vi "QMH Main.vi"() -> ()   [LabVIEW 2021]
doc: "Demonstrates the fundamentals of the Queued Message Handler design pattern in LabVIEW. A queued message handler, in its simplest form, is composed of two loops. The Event Handling Loop responds to user interface events by enqueuing \"messages\" on a message queue. These messages are dequeued in the Message Handling Loop. Note that the Message Handling Loop is also capable of sending messages to itself."
uses:
  <vilib>/MakerHub/PS4-Controller/Private/Type Defs/Indicators/Controller.ctl
  <vilib>/MakerHub/PS4-Controller/Private/Type Defs/Indicators/Square.ctl
  <vilib>/MakerHub/PS4-Controller/Private/Type Defs/Indicators/X.ctl
  <vilib>/MakerHub/PS4-Controller/Private/Type Defs/Indicators/Circle.ctl
  <vilib>/MakerHub/PS4-Controller/Private/Type Defs/Indicators/Triangle.ctl
  <vilib>/MakerHub/PS4-Controller/Private/Type Defs/Indicators/L1.ctl
  <vilib>/MakerHub/PS4-Controller/Private/Type Defs/Indicators/R1.ctl
  <vilib>/MakerHub/PS4-Controller/Private/Type Defs/Indicators/Share.ctl
  <vilib>/MakerHub/PS4-Controller/Private/Type Defs/Indicators/Options.ctl
  <vilib>/MakerHub/PS4-Controller/Private/Type Defs/Indicators/PS.ctl
  <vilib>/MakerHub/PS4-Controller/Private/Type Defs/Indicators/Pad_Button.ctl
  <vilib>/MakerHub/PS4-Controller/Private/Type Defs/Indicators/Dpad.ctl
  <vilib>/MakerHub/PS4-Controller/Private/Type Defs/Indicators/Slider.ctl
  C:/Program Files (x86)/National Instruments/LabVIEW 2021/examples/Design Patterns/Queued Message Handler/support/QMH Fundamentals - Message Cluster.ctl
  Classes/Actuation/Spring Motor/Spring Motor.lvclass
  Classes/Actuation/Motor/DC Motor.lvclass
  Classes/Sensing/IMU/IMU.lvclass
  Classes/Sensing/Ultrasonic Sensor/Ultrasonic Sensor.lvclass
  <vilib>/Utility/error.llb/Error Cluster From Error Code.vi
  <vilib>/MakerHub/PS4-Controller/Public/Open First Controller.vi
  <vilib>/ErrorRing/Error Ring.xnode
  Classes/Communication/Comm/Comm.lvclass
  <vilib>/MakerHub/PS4-Controller/LMH-PS4.lvlib
panel:
  out "PS4 Controller":T1={"Square Button"=FALSE, "X Button"=FALSE, "Circle Button"=FALSE, "Triangle Button"=FALSE, "L1"=FALSE, "R1"=FALSE, "Share Button"=FALSE, "Options Button"=FALSE, "PS Button"=FALSE, "Pad Button"=FALSE, "D-Pad"=5, "L2"=0, "R2"=0, "Thumbstick_Left"={[], []}, "Thumbstick_Right"={[], []}} {"R2" scale=-32768.0..32767.0; "L2" scale=-32768.0..32767.0}
  out "Checkbox":bool
  out "error out":errorcluster
  in  "Motor B Enable":bool
  in  "Motor B PWM":i16(slide) scale=0.0..255.0
  in  "Motor A Enable":bool
  in  "Motor A PWM":i16(slide) scale=0.0..255.0
  in  "Spring Motor Enable":bool
  in  "Spring Motor PWM":i16(slide) scale=0.0..180.0
  out "Display Message":string
  in  "Stop":bool
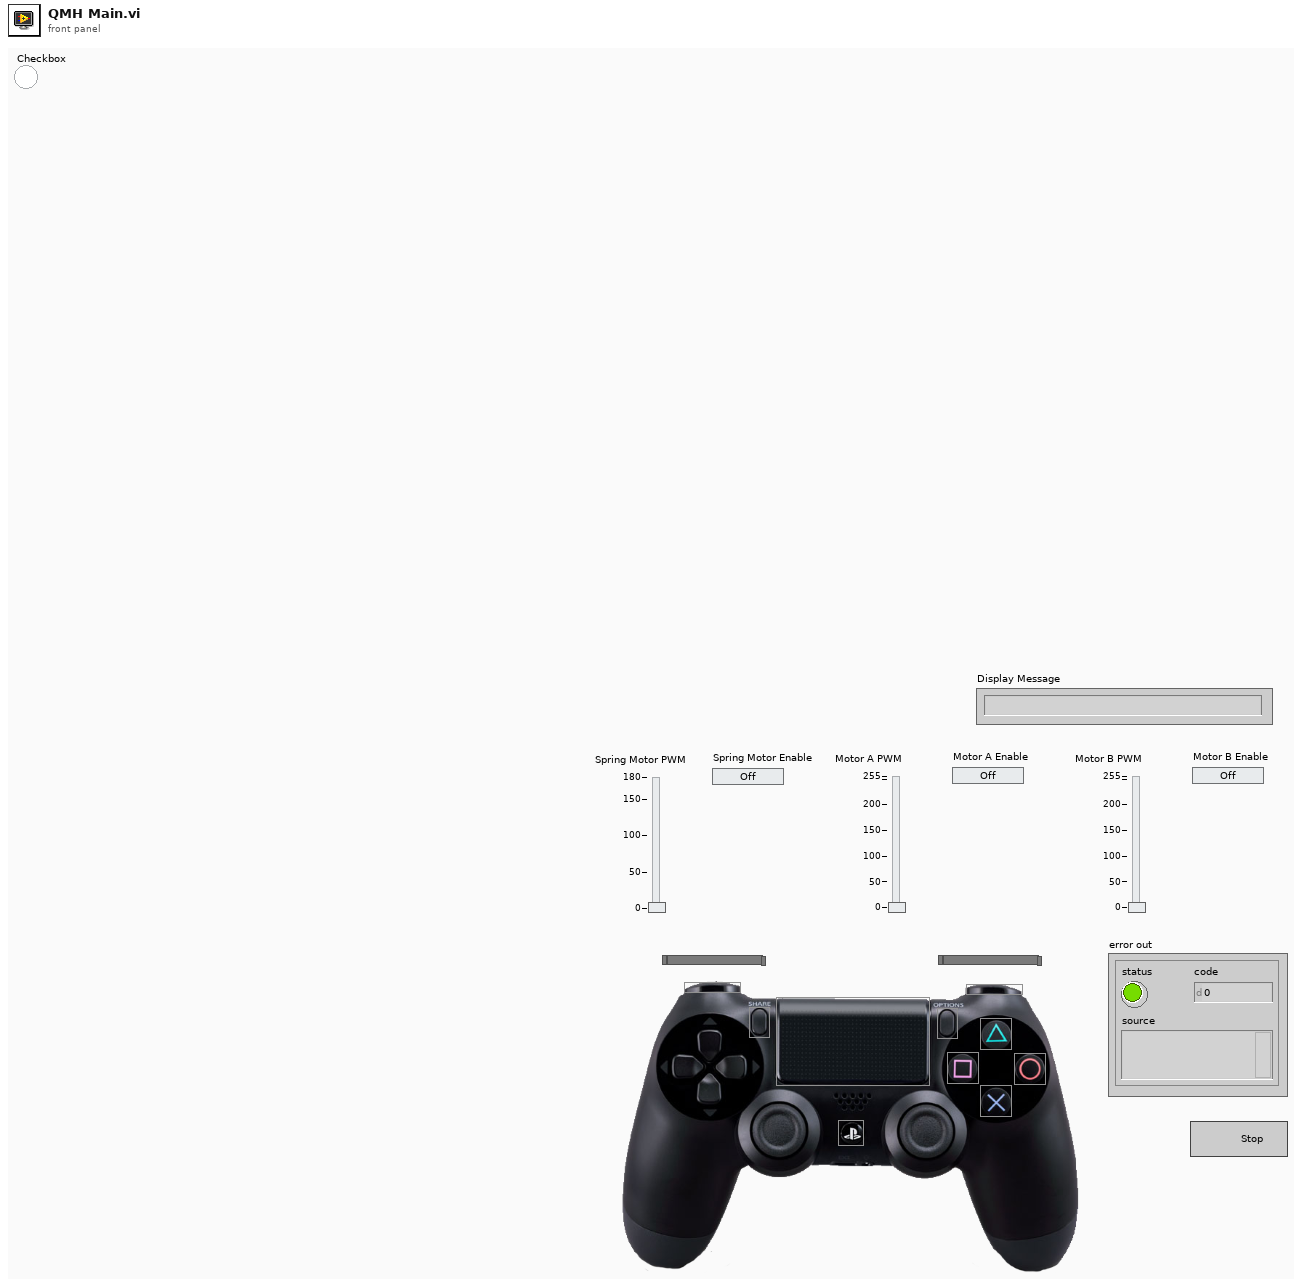
[diagram p1: front panel]
types:
  T1 = typedef "LMH-PS4.lvlib/Controller.ctl" = cluster{"Square Button":T2, "X Button":T3, "Circle Button":T4, "Triangle Button":T5, "L1":T6, "R1":T7, "Share Button":T8, "Options Button":T9, "PS Button":T10, "Pad Button":T11, "D-Pad":T12, "L2":T13, "R2":T13, "Thumbstick_Left":cluster{i32[], i32[]}, "Thumbstick_Right":cluster{i32[], i32[]}}
  T2 = typedef "LMH-PS4.lvlib/Square.ctl" = bool
  T3 = typedef "LMH-PS4.lvlib/X.ctl" = bool
  T4 = typedef "LMH-PS4.lvlib/Circle.ctl" = bool
  T5 = typedef "LMH-PS4.lvlib/Triangle.ctl" = bool
  T6 = typedef "LMH-PS4.lvlib/L1.ctl" = bool
  T7 = typedef "LMH-PS4.lvlib/R1.ctl" = bool
  T8 = typedef "LMH-PS4.lvlib/Share.ctl" = bool
  T9 = typedef "LMH-PS4.lvlib/Options.ctl" = bool
  T10 = typedef "LMH-PS4.lvlib/PS.ctl" = bool
  T11 = typedef "LMH-PS4.lvlib/Pad_Button.ctl" = bool
  T12 = typedef "LMH-PS4.lvlib/Dpad.ctl" = u16
  T13 = typedef "LMH-PS4.lvlib/Slider.ctl" = i32
  T14 = typedef "QMH Fundamentals - Message Cluster.ctl" = cluster{"Message":string, "Message Data":variant}
  T15 = typedef "LMH-PS4.lvlib/PS4 Controller Ref.ctl" = cluster{"Controller Ref":refnum<k1>, "Worker Ref":refnum<vi>, "PS4 Events Ref":refnum<event-registration>}
  T16 = typedef "LMH-PS4.lvlib/Axis.ctl" = cluster{"Left Thumbstick":cluster{"X Axis":i32, "Y Axis":i32}, "Right Thumbstick":cluster{"X Axis":i32, "Y Axis":i32}, "L2":i32, "R2":i32, "D-Pad":T17}
  T17 = typedef "LMH-PS4.lvlib/DPad Enum.ctl" = enum16{"Idle", "Up", "Up / Right", "Right", "Down / Right", "Down", "Down / Left", "Left", "Up / Left"}
  T18 = typedef "LMH-PS4.lvlib/Buttons.ctl" = cluster{"Square":bool, "X":bool, "Circle":bool, "Triangle":bool, "L1":bool, "R1":bool, "L2":bool, "R2":bool, "Share":bool, "Options":bool, "Left Thumbstick":bool, "Right Thumbstick":bool, "Playstation Button":bool, "Pad":bool}
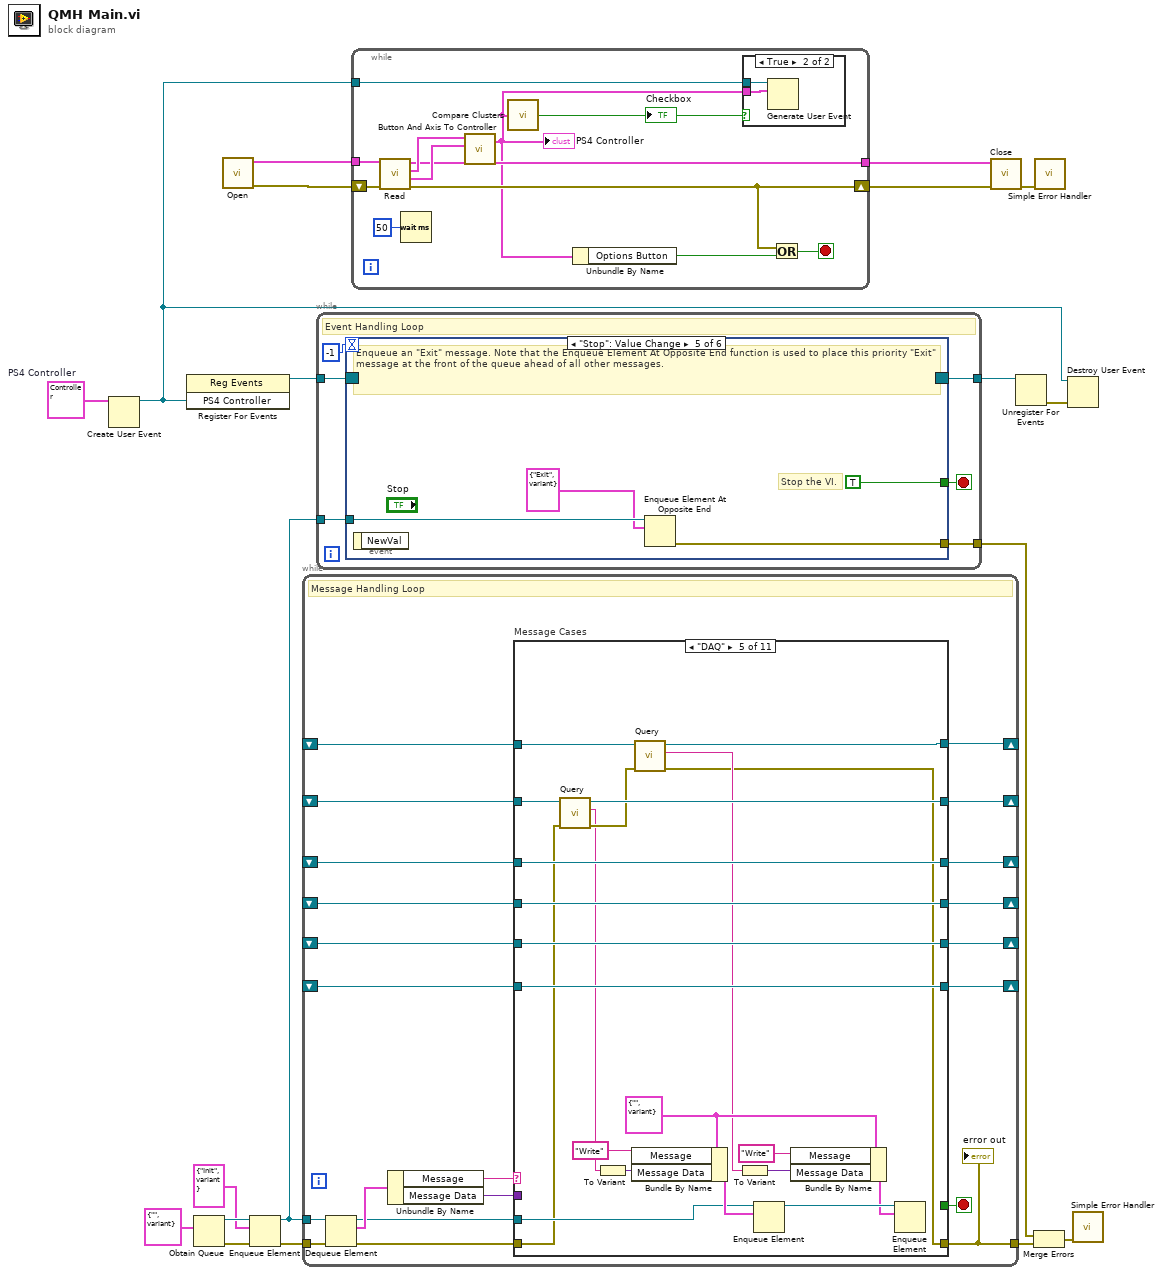
[diagram p0: block diagram]
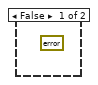
[diagram p2: hidden frame]
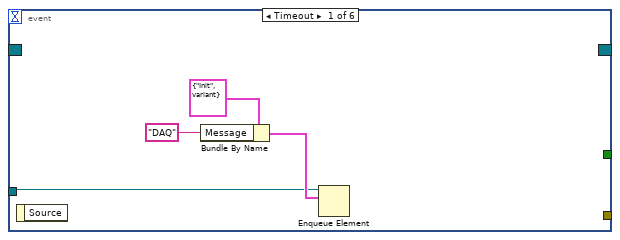
[diagram p3: hidden frame]
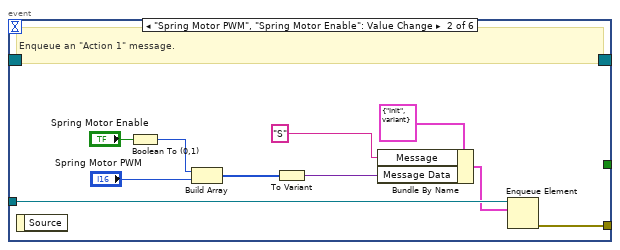
[diagram p4: hidden frame]
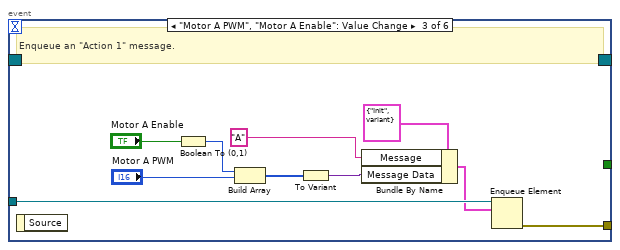
[diagram p5: hidden frame]
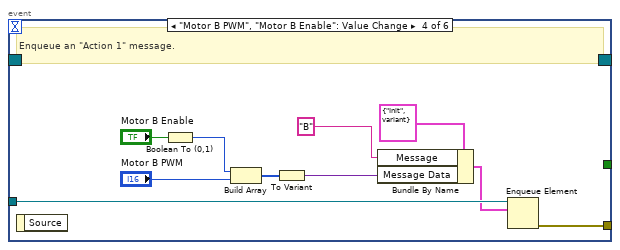
[diagram p6: hidden frame]
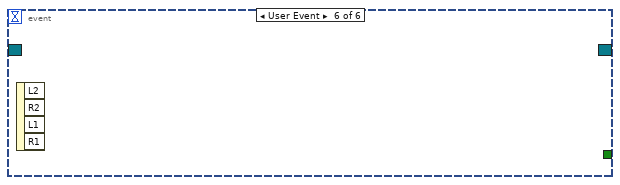
[diagram p7: hidden frame]
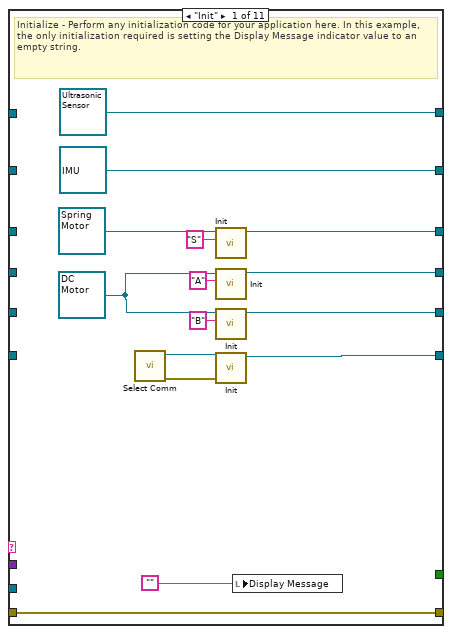
[diagram p8: hidden frame]
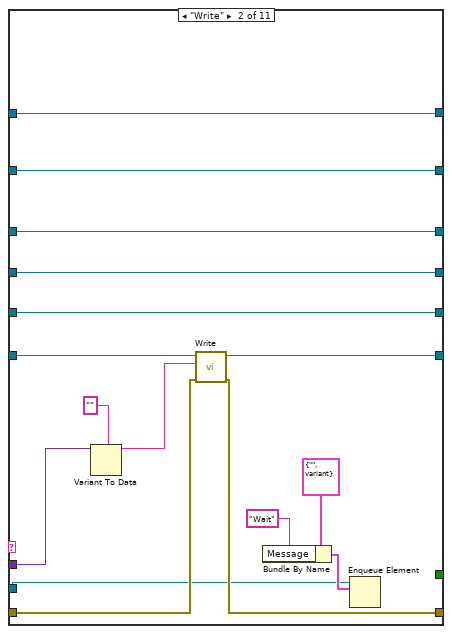
[diagram p9: hidden frame]
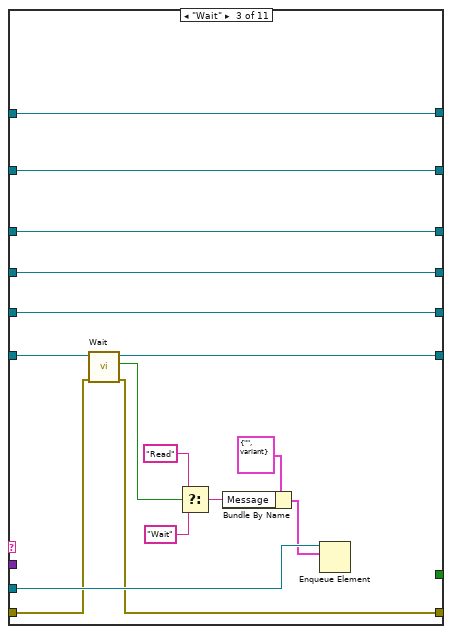
[diagram p10: hidden frame]
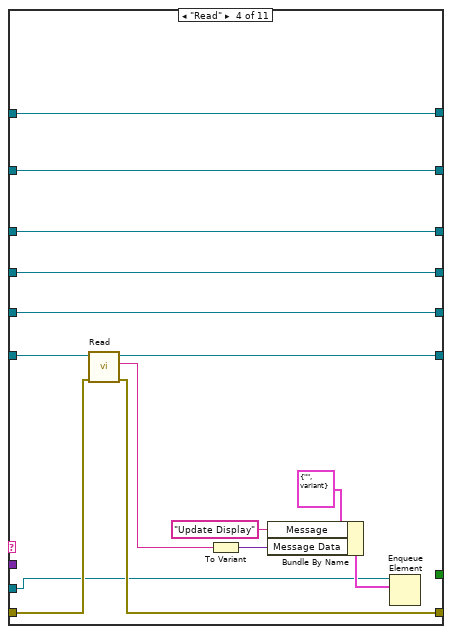
[diagram p11: hidden frame]
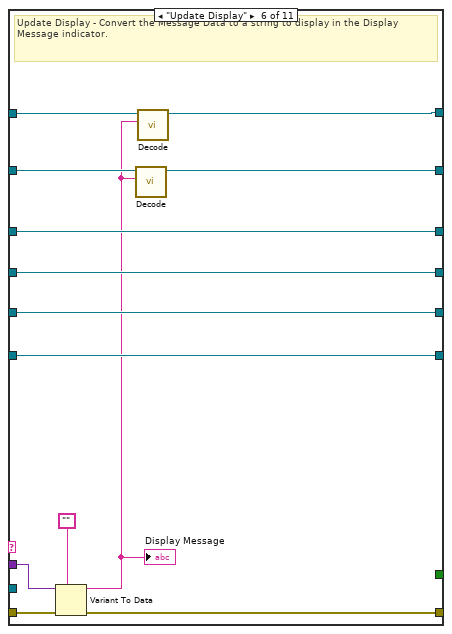
[diagram p12: hidden frame]
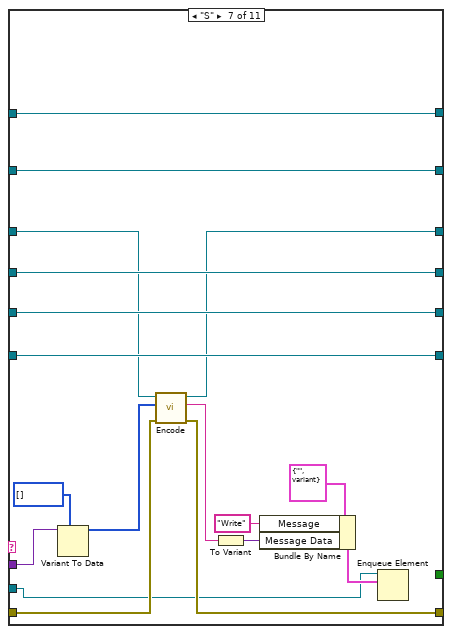
[diagram p13: hidden frame]
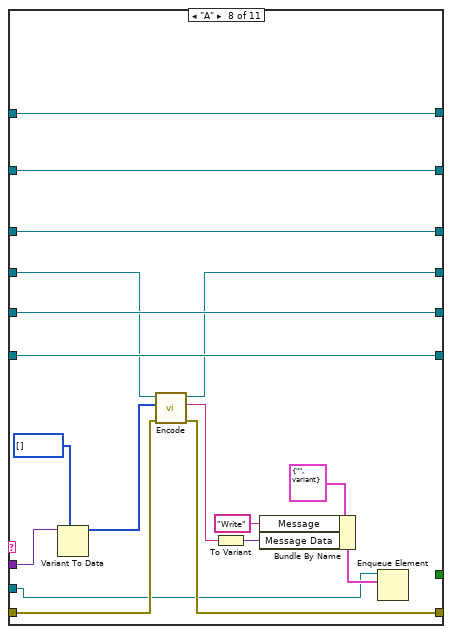
[diagram p14: hidden frame]
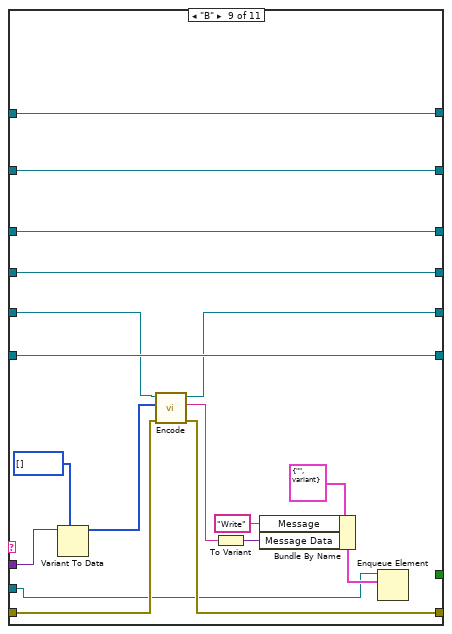
[diagram p15: hidden frame]
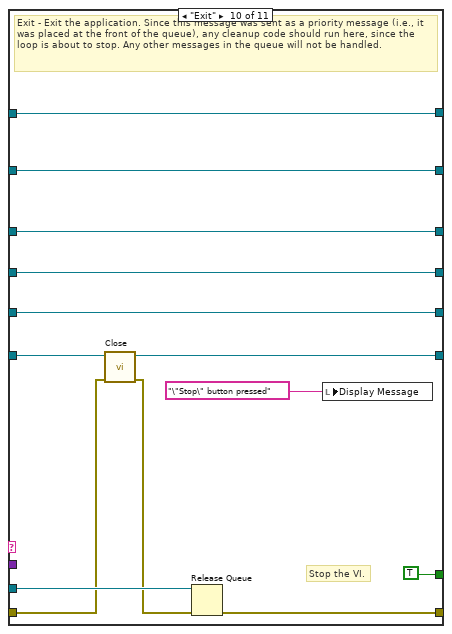
[diagram p16: hidden frame]
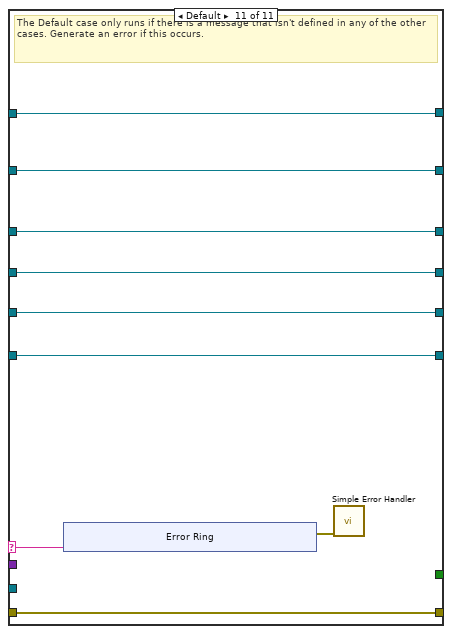
[diagram p17: hidden frame]
diagram:
  w5 = T1 {"Square Button"=FALSE, "X Button"=FALSE, "Circle Button"=FALSE, "Triangle Button"=FALSE, "L1"=FALSE, "R1"=FALSE, "Share Button"=FALSE, "Options Button"=FALSE, "PS Button"=FALSE, "Pad Button"=FALSE, "D-Pad"=5, "L2"=0, "R2"=0, "Thumbstick_Left"={[], []}, "Thumbstick_Right"={[], []}}  # PS4 Controller
  n1 = Create User Event(user event datatype=w5) -> (user event=w1:refnum<user-event>)  [unwired: 1 in, 1 out]
  n2 = register-events(w1) -> (reference out=w4:refnum<event-registration>)  [unwired: 2 in, 1 out]
  n3 = Obtain Queue(element data type=T14 {"Message"="", "Message Data"=variant} ("Message Cluster")) -> (queue out=w15:refnum<queue>, error out=w16:errorcluster)  [unwired: 4 in, 1 out]
  n4 = call-poly <vilib>:"Open.vi"() -> ("Error Out"=w7:errorcluster, "PS4 Controller Ref"=w6:T15)  [unwired: 9 in, 1 out]
  n5 = Enqueue Element(queue=w15, element=T14 {"Message"="Init", "Message Data"=variant}, error in (no error)=w16) -> (queue out=w13:refnum<queue>, error out=w14:errorcluster)  [unwired: 1 in, 1 out]
  n6 = while {
    tunnel: w13 -> [w37]
    tunnel: w14 -> [w38]
    tunnel: [w39] -> w19
    shift-right: [w31] -> _
    shift-left: _ -> [w27]
    shift-right: [w28] -> _
    shift-left: _ -> [w24]
    shift-right: [w29] -> _
    shift-left: _ -> [w25]
    shift-right: [w30] -> _
    shift-left: _ -> [w26]
    shift-right: [w23] -> _
    shift-left: _ -> [w22]
    shift-right: [w21] -> _
    shift-left: _ -> [w20]
    stop <- w40 stop-if-true
    # "Message Handling Loop"
    n7 = Dequeue Element(queue=w37, error in (no error)=w38) -> (queue out=w35:refnum<queue>, element=w36:T14, error out=w34:errorcluster)  [unwired: 1 in, 1 out]
    n8 = Unbundle By Name(w36) -> ("Message"=w33:string, "Message Data"=w32:variant)
    n9 = case "Message Cases" shown="\"DAQ\"" w33 {
      selector: w33 -> [_ _ _ _ _ _ _ _ _ _ w213]
      tunnel: w35 -> [_ w61 w81 w93 w115 _ w141 w163 w180 w204 _]
      tunnel: w34 -> [w55 w63 w80 w97 w107 w137 w143 w165 w182 w197 w212]
      tunnel: [w55 w62 w79 w96 w103 w134 w142 w164 w181 w202 w212] -> w39
      tunnel: [_ _ _ _ _ _ _ _ _ TRUE _] -> w40
      tunnel: w32 -> [_ w69 _ _ _ w136 w150 w172 w189 _ _]
      tunnel: [w51 w70 w83 w98 w124 w130 w153 w173 w190 w194 w207] -> w31
      tunnel: [w47 w60 w87 w102 w123 w133 w151 w162 w178 w200 w210] -> w30
      tunnel: [w46 w59 w86 w101 w122 w132 w155 w159 w191 w199 w209] -> w29
      tunnel: [w45 w58 w85 w100 w121 w131 w154 w161 w177 w198 w208] -> w28
      tunnel: w27 -> [_ w71 w84 w99 w124 w130 w153 w173 w190 w195 w207]
      tunnel: w26 -> [_ w60 w87 w102 w123 w133 w152 w162 w178 w200 w210]
      tunnel: w25 -> [_ w59 w86 w101 w122 w132 w155 w160 w191 w199 w209]
      tunnel: w24 -> [_ w58 w85 w100 w121 w131 w154 w161 w179 w198 w208]
      tunnel: [refnum<class "IMU.lvclass"> refnum ("IMU.lvclass") w57 w73 w89 w109 w127 w140 w158 w176 w193 w206] -> w23
      tunnel: w22 -> [_ w57 w73 w89 w120 w129 w140 w158 w176 w193 w206]
      tunnel: [refnum<class "Ultrasonic Sensor.lvclass"> refnum ("Ultrasonic Sensor.lvclass") w56 w72 w88 w108 w126 w139 w157 w175 w192 w205] -> w21
      tunnel: w20 -> [_ w56 w72 w88 w119 w128 w139 w157 w175 w192 w205]
      frame "Init" {
        w43 = refnum<class "DC Motor.lvclass"> refnum ("DC Motor.lvclass")
        # "Initialize - Perform any initialization code for your application here. In this example, the only initialization required is setting the Display Message indicator value to an empty string."
        n10 = call "Select Comm.vi"() -> ("error out"=w52:errorcluster, "Comm.lvclass"=w53:refnum<class "Comm.lvclass">)  [unwired: 10 in]
        n11 = call-dynamic "Init.vi"("ID"="S", "Spring Motor in"=refnum<class "Spring Motor.lvclass"> refnum) -> ("Spring Motor out"=w47:refnum<class "Spring Motor.lvclass">)  [unwired: 8 in, 1 out]
        n12 = call-dynamic "Init.vi"("ID"="A", "DC Motor in"=w43) -> ("DC Motor out"=w46:refnum<class "DC Motor.lvclass">)  [unwired: 8 in, 1 out]
        n13 = call-dynamic "Init.vi"("ID"="B", "DC Motor in"=w43) -> ("DC Motor out"=w45:refnum<class "DC Motor.lvclass">)  [unwired: 8 in, 1 out]
        n14 = call-dynamic "Init.vi"("error in (no error)"=w52, "Comm in"=w53) -> ("Comm out"=w51:refnum<class "Comm.lvclass">)  [unwired: 8 in, 1 out]
        n15 = local write "Display Message"("") -> ()
      }
      frame "Write" {
        n16 = Variant To Data(type="", Variant=w69) -> (data=w67:string)  [unwired: 1 in, 1 out]
        n17 = call-dynamic "Write.vi"("error in (no error)"=w63, "Message"=w67, "Comm in"=w71) -> ("error out"=w62:errorcluster, "Comm out"=w70:refnum<class "Comm.lvclass">)  [unwired: 7 in]
        n18 = Bundle By Name(cluster=T14 {"Message"="", "Message Data"=variant} ("Message Cluster"), "Message"="Wait") -> (w66:T14)
        n19 = Enqueue Element(queue=w61, element=w66) -> ()  [unwired: 2 in, 3 out]
      }
      frame "Wait" {
        n20 = call-dynamic "Wait.vi"("error in (no error)"=w80, "Comm in"=w84) -> ("error out"=w79:errorcluster, "Ready?"=w78:bool, "Comm out"=w83:refnum<class "Comm.lvclass">)  [unwired: 7 in]
        n21 = Select(t="Read" ("Message"), s=w78, f="Wait" ("Message")) -> (s? t:f=w75:string)
        n22 = Bundle By Name(cluster=T14 {"Message"="", "Message Data"=variant} ("Message Cluster"), "Message"=w75) -> (w74:T14)
        n23 = Enqueue Element(queue=w81, element=w74) -> ()  [unwired: 2 in, 3 out]
      }
      frame "Read" {
        n24 = call-dynamic <vilib>:"Read.vi"("error in (no error)"=w97, "Comm in"=w99) -> ("error out"=w96:errorcluster, "Message"=w91:string, "Comm out"=w98:refnum<class "Comm.lvclass">)  [unwired: 7 in]
        n25 = To Variant(anything=w91) -> (Variant=w92:variant)
        n26 = Bundle By Name(cluster=T14 {"Message"="", "Message Data"=variant} ("Message Cluster"), "Message"="Update Display", "Message Data"=w92) -> (w95:T14)
        n27 = Enqueue Element(queue=w93, element=w95) -> ()  [unwired: 2 in, 3 out]
      }
      frame "DAQ" {
        w111 = T14 {"Message"="", "Message Data"=variant} ("Message Cluster")
        n28 = call-dynamic "Query.vi"("error in (no error)"=w107, "IMU in"=w120) -> ("error out"=w106:errorcluster, "Message"=w105:string, "IMU out"=w109:refnum<class "IMU.lvclass">)  [unwired: 7 in]
        n29 = To Variant(anything=w105) -> (Variant=w117:variant)
        n30 = Bundle By Name(cluster=w111, "Message"="Write", "Message Data"=w117) -> (w118:T14)
        n31 = call-dynamic "Query.vi"("error in (no error)"=w106, "Ultrasonic Sensor in"=w119) -> ("error out"=w103:errorcluster, "Message"=w104:string, "Ultrasonic Sensor out"=w108:refnum<class "Ultrasonic Sensor.lvclass">)  [unwired: 7 in]
        n32 = To Variant(anything=w104) -> (Variant=w113:variant)
        n33 = Enqueue Element(queue=w115, element=w118) -> (queue out=w112:refnum<queue>)  [unwired: 2 in, 2 out]
        n34 = Bundle By Name(cluster=w111, "Message"="Write", "Message Data"=w113) -> (w110:T14)
        n35 = Enqueue Element(queue=w112, element=w110) -> ()  [unwired: 2 in, 3 out]
      }
      frame "Update Display" {
        # "Update Display - Convert the Message Data to a string to display in the Display Message indicator."
        n36 = Variant To Data(error in=w137, type="", Variant=w136) -> (data=w125:string, error out=w134:errorcluster)
        "Display Message" <- w125
        n37 = call-dynamic "Decode.vi"("Input String"=w125, "IMU in"=w129) -> ("IMU out"=w127:refnum<class "IMU.lvclass">)  [unwired: 8 in, 1 out]
        n38 = call-dynamic "Decode.vi"("Message in"=w125, "Ultrasonic Sensor in"=w128) -> ("Ultrasonic Sensor out"=w126:refnum<class "Ultrasonic Sensor.lvclass">)  [unwired: 8 in, 1 out]
      }
      frame "S" {
        n39 = Variant To Data(type=i16[] [] ("appended array"), Variant=w150) -> (data=w149:i16[])  [unwired: 1 in, 1 out]
        n40 = call-dynamic "Encode.vi"("error in (no error)"=w143, "Data"=w149, "Spring Motor in"=w152) -> ("error out"=w142:errorcluster, "Message"=w145:string, "Spring Motor out"=w151:refnum<class "Spring Motor.lvclass">)  [unwired: 6 in]
        n41 = To Variant(anything=w145) -> (Variant=w144:variant)
        n42 = Bundle By Name(cluster=T14 {"Message"="", "Message Data"=variant} ("Message Cluster"), "Message"="Write", "Message Data"=w144) -> (w148:T14)
        n43 = Enqueue Element(queue=w141, element=w148) -> ()  [unwired: 2 in, 3 out]
      }
      frame "A" {
        n44 = Variant To Data(type=i16[] [] ("appended array"), Variant=w172) -> (data=w171:i16[])  [unwired: 1 in, 1 out]
        n45 = call-dynamic "Encode.vi"("error in (no error)"=w165, "Data"=w171, "DC Motor in"=w160) -> ("error out"=w164:errorcluster, "Message"=w167:string, "DC Motor out"=w159:refnum<class "DC Motor.lvclass">)  [unwired: 6 in]
        n46 = To Variant(anything=w167) -> (Variant=w166:variant)
        n47 = Bundle By Name(cluster=T14 {"Message"="", "Message Data"=variant} ("Message Cluster"), "Message"="Write", "Message Data"=w166) -> (w170:T14)
        n48 = Enqueue Element(queue=w163, element=w170) -> ()  [unwired: 2 in, 3 out]
      }
      frame "B" {
        n49 = Variant To Data(type=i16[] [] ("appended array"), Variant=w189) -> (data=w188:i16[])  [unwired: 1 in, 1 out]
        n50 = call-dynamic "Encode.vi"("error in (no error)"=w182, "Data"=w188, "DC Motor in"=w179) -> ("error out"=w181:errorcluster, "Message"=w184:string, "DC Motor out"=w177:refnum<class "DC Motor.lvclass">)  [unwired: 6 in]
        n51 = To Variant(anything=w184) -> (Variant=w183:variant)
        n52 = Bundle By Name(cluster=T14 {"Message"="", "Message Data"=variant} ("Message Cluster"), "Message"="Write", "Message Data"=w183) -> (w187:T14)
        n53 = Enqueue Element(queue=w180, element=w187) -> ()  [unwired: 2 in, 3 out]
      }
      frame "Exit" {
        # "Stop the VI."
        # "Exit - Exit the application. Since this message was sent as a priority message (i.e., it was placed at the front of the queue), any cleanup code should run here, since the loop is about to stop. Any other messages in the queue will not be handled."
        n54 = call-dynamic <vilib>:"Close.vi"("error in (no error)"=w197, "Comm in"=w195) -> ("error out"=w196:errorcluster, "Comm out"=w194:refnum<class "Comm.lvclass">)  [unwired: 8 in]
        n55 = Release Queue(queue=w204, error in (no error)=w196) -> (error out=w202:errorcluster)  [unwired: 1 in, 2 out]
        n56 = local write "Display Message"("\"Stop\" button pressed" ("L10n_Stop Pressed")) -> ()
      }
      frame Default {
        # "The Default case only runs if there is a message that isn't defined in any of the other cases. Generate an error if this occurs."
        n57 = xnode "Error Ring"("parameter 0"=w213) -> ("error out"=w211:errorcluster)
        n58 = call <vilib>:"Simple Error Handler.vi"("error in (no error)"=w211) -> ()  [unwired: 4 in, 5 out]
      }
    }
    "error out" <- w39
  }
  n59 = while {
    tunnel: w13 -> [w226]
    tunnel: [w224] -> w18
    tunnel: w4 -> [w222]
    tunnel: [w221] -> w2
    stop <- w225 stop-if-true
    # "Event Handling Loop"
    n60 = event shown="[4] \"Stop\": Value Change" {
      selector: w222 -> [_ _ _ _ _ _]
      dyn-events: [_ _ _ _ _ _] -> w221
      timeout: -1 -> [_ _ _ _ _ _]
      tunnel: [_ _ _ _ TRUE _] -> w225
      tunnel: w226 -> [w228 w240 w250 w260 w264 _]
      tunnel: [_ w239 w249 w259 w263 _] -> w224
      event Timeout {
        n61 = event-data() -> ()  [unwired: 1 in, 1 out]
        n62 = Bundle By Name(cluster=T14 {"Message"="Init", "Message Data"=variant} ("element"), "Message"="DAQ") -> (w229:T14)
        n63 = Enqueue Element(queue=w228, element=w229) -> ()  [unwired: 2 in, 3 out]
      }
      event "Spring Motor PWM", "Spring Motor Enable": Value Change {
        # "Enqueue an \"Action 1\" message."
        n64 = event-data() -> ()  [unwired: 1 in, 1 out]
        n65 = Boolean To (0,1)(Boolean="Spring Motor Enable") -> (0, 1=w231:i16)
        n66 = Build Array(w231, "Spring Motor PWM") -> (w233:i16[])
        n67 = To Variant(anything=w233) -> (Variant=w235:variant)
        n68 = Bundle By Name(cluster=T14 {"Message"="Init", "Message Data"=variant} ("element"), "Message"="S", "Message Data"=w235) -> (w237:T14)
        n69 = Enqueue Element(queue=w240, element=w237) -> (error out=w239:errorcluster)  [unwired: 2 in, 2 out]
      }
      event "Motor A PWM", "Motor A Enable": Value Change {
        # "Enqueue an \"Action 1\" message."
        n70 = event-data() -> ()  [unwired: 1 in, 1 out]
        n71 = Boolean To (0,1)(Boolean="Motor A Enable") -> (0, 1=w242:i16)
        n72 = Build Array(w242, "Motor A PWM") -> (w244:i16[])
        n73 = To Variant(anything=w244) -> (Variant=w246:variant)
        n74 = Bundle By Name(cluster=T14 {"Message"="Init", "Message Data"=variant} ("element"), "Message"="A", "Message Data"=w246) -> (w247:T14)
        n75 = Enqueue Element(queue=w250, element=w247) -> (error out=w249:errorcluster)  [unwired: 2 in, 2 out]
      }
      event "Motor B PWM", "Motor B Enable": Value Change {
        # "Enqueue an \"Action 1\" message."
        n76 = event-data() -> ()  [unwired: 1 in, 1 out]
        n77 = Boolean To (0,1)(Boolean="Motor B Enable") -> (0, 1=w251:i16)
        n78 = Build Array(w251, "Motor B PWM") -> (w253:i16[])
        n79 = To Variant(anything=w253) -> (Variant=w256:variant)
        n80 = Bundle By Name(cluster=T14 {"Message"="Init", "Message Data"=variant} ("element"), "Message"="B", "Message Data"=w256) -> (w257:T14)
        n81 = Enqueue Element(queue=w260, element=w257) -> (error out=w259:errorcluster)  [unwired: 2 in, 2 out]
      }
      event "Stop": Value Change {
        # "Stop the VI."
        # "Enqueue an \"Exit\" message. Note that the Enqueue Element At Opposite End function is used to place this priority \"Exit\" message at the front of the queue ahead of all other messages."
        n82 = event-data() -> ()  [unwired: 1 in, 1 out]
        n83 = Enqueue Element At Opposite End(queue=w264, element=T14 {"Message"="Exit", "Message Data"=variant}) -> (error out=w263:errorcluster)  [unwired: 2 in, 2 out]
      }
      event User Event {
        n84 = event-data() -> ()  [unwired: 1 in, 4 out]
      }
    }
  }
  n85 = while {
    shift-right: [w273] -> w10
    shift-left: w7 -> [w270]
    tunnel: [w272] -> w8
    tunnel: w6 -> [w271]
    tunnel: w1 -> [w265]
    stop <- w274 stop-if-true
    n86 = call <vilib>:"Read.vi"("Error In"=w270, "PS4 Controller Ref"=w271) -> ("Error Out"=w273:errorcluster, "All Axis"=w276:T16, "Buttons"=w275:T18, "PS4 Controller Ref"=w272:T15)  [unwired: 6 in]
    n87 = Wait (ms)(milliseconds to wait=u32 50) -> ()  [unwired: 1 out]
    n88 = call <vilib>:"Button And Axis To Controller.vi"("All Axis"=w276, "Buttons"=w275) -> ("PS4 Controller"=w267:T1)  [unwired: 5 in]
    "PS4 Controller" <- w267
    n89 = call "Compare Clusters.vi"("PS4 Controller"=w267) -> ("Checkbox"=w268:bool)
    "Checkbox" <- w268
    n90 = Unbundle By Name(w267) -> ("Options Button"=w266:T9)
    n91 = case shown="True" w268 {
      tunnel: w267 -> [_ w278]
      tunnel: w265 -> [_ w277]
      frame False {
        (unwired) errorcluster {"status"=FALSE, "code"=0, "source"=""} ("error out")
      }
      frame True {
        n92 = Generate User Event(user event=w277, event data cluster=w278) -> ()  [unwired: 2 in, 2 out]
      }
    }
    n93 = Or(x=w273, y=w266) -> (x .or. y?=w274:T9)
  }
  n94 = call <vilib>:"Close.vi"("Error In"=w10, "PS4 Controller Ref"=w8) -> ("Error Out"=w9:errorcluster)  [unwired: 9 in]
  n95 = Unregister For Events(event registration refnum=w2) -> (error out=w3:errorcluster)  [unwired: 1 in]
  n96 = Merge Errors(w18, w19) -> (w11:errorcluster)
  n97 = call <vilib>:"Simple Error Handler.vi"("error in (no error)"=w9) -> ()  [unwired: 4 in, 5 out]
  n98 = Destroy User Event(user event=w1, error in=w3) -> ()  [unwired: 1 out]
  n99 = call <vilib>:"Simple Error Handler.vi"("error in (no error)"=w11) -> ()  [unwired: 4 in, 5 out]
